vi "Simulator.vi"() -> ()   [LabVIEW 2018]
uses:
  Commands/Address.ctl
  <vilib>/FPGAPlugInAG/cRIO-9039/niLvFpga_Open_cRIO-9039.vi
  <vilib>/rvi/interface/common/dynamic/niFpgaDynamicAddResources.vi
  <vilib>/Utility/error.llb/Error Cluster From Error Code.vi
  <vilib>/rvi/errors/niLvFpgaAdjustHostInterfaceError.vi
  <vilib>/FPGAPlugInAG/Dynamic/niLvFpga_Close_Dynamic.vi
  <vilib>/rvi/interface/nirviOpenFPGA/nirviOpenFPGA.xnode
  FPGA Bitfiles/M1M3SupportSimulator.lvbitx
  <vilib>/rvi/interface/nirviMethod/nirviMethod.xnode
  <vilib>/rvi/interface/nirviCloseFPGA/nirviCloseFPGA.xnode
  <vilib>/rvi/errors/niLvFpgaMergeErrorWithErrorCode.vi
  <vilib>/FPGAPlugInAG/Dynamic/niLvFpga_WriteFifo_Dynamic.vi
  <vilib>/FPGAPlugInAG/Dynamic/niLvFpga_ReadFifo_Dynamic.vi
panel:
  out "E Instr":u64
  out "E Flags":u64 format="%04x"
  out "ERx":u64
  out "ETx":u64
  out "D Instr":u64
  out "D Flags":u64 format="%04x"
  out "DRx":u64
  out "DTx":u64
  out "C Instr":u64
  out "C Flags":u64 format="%04x"
  out "CRx":u64
  out "CTx":u64
  out "B Instr":u64
  out "B Flags":u64 format="%04x"
  out "BRx":u64
  out "BTx":u64
  out "String 5":string
  out "String 4":string
  out "String 3":string
  out "String 2":string
  out "String":string
  in  "Process Stop Button":bool
  out "A Instr":u64
  out "A Flags":u64 format="%04x"
  out "Error":string
  out "Loop count":dbl
  out "ARx":u64
  out "ATx":u64
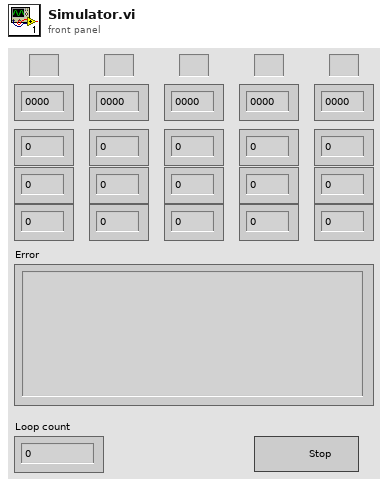
[diagram p1: front panel]
types:
  T1 = typedef "Address.ctl" = enum16{"ModbusA", "ModbusB", "ModbusC", "ModbusD", "ModbusE"}
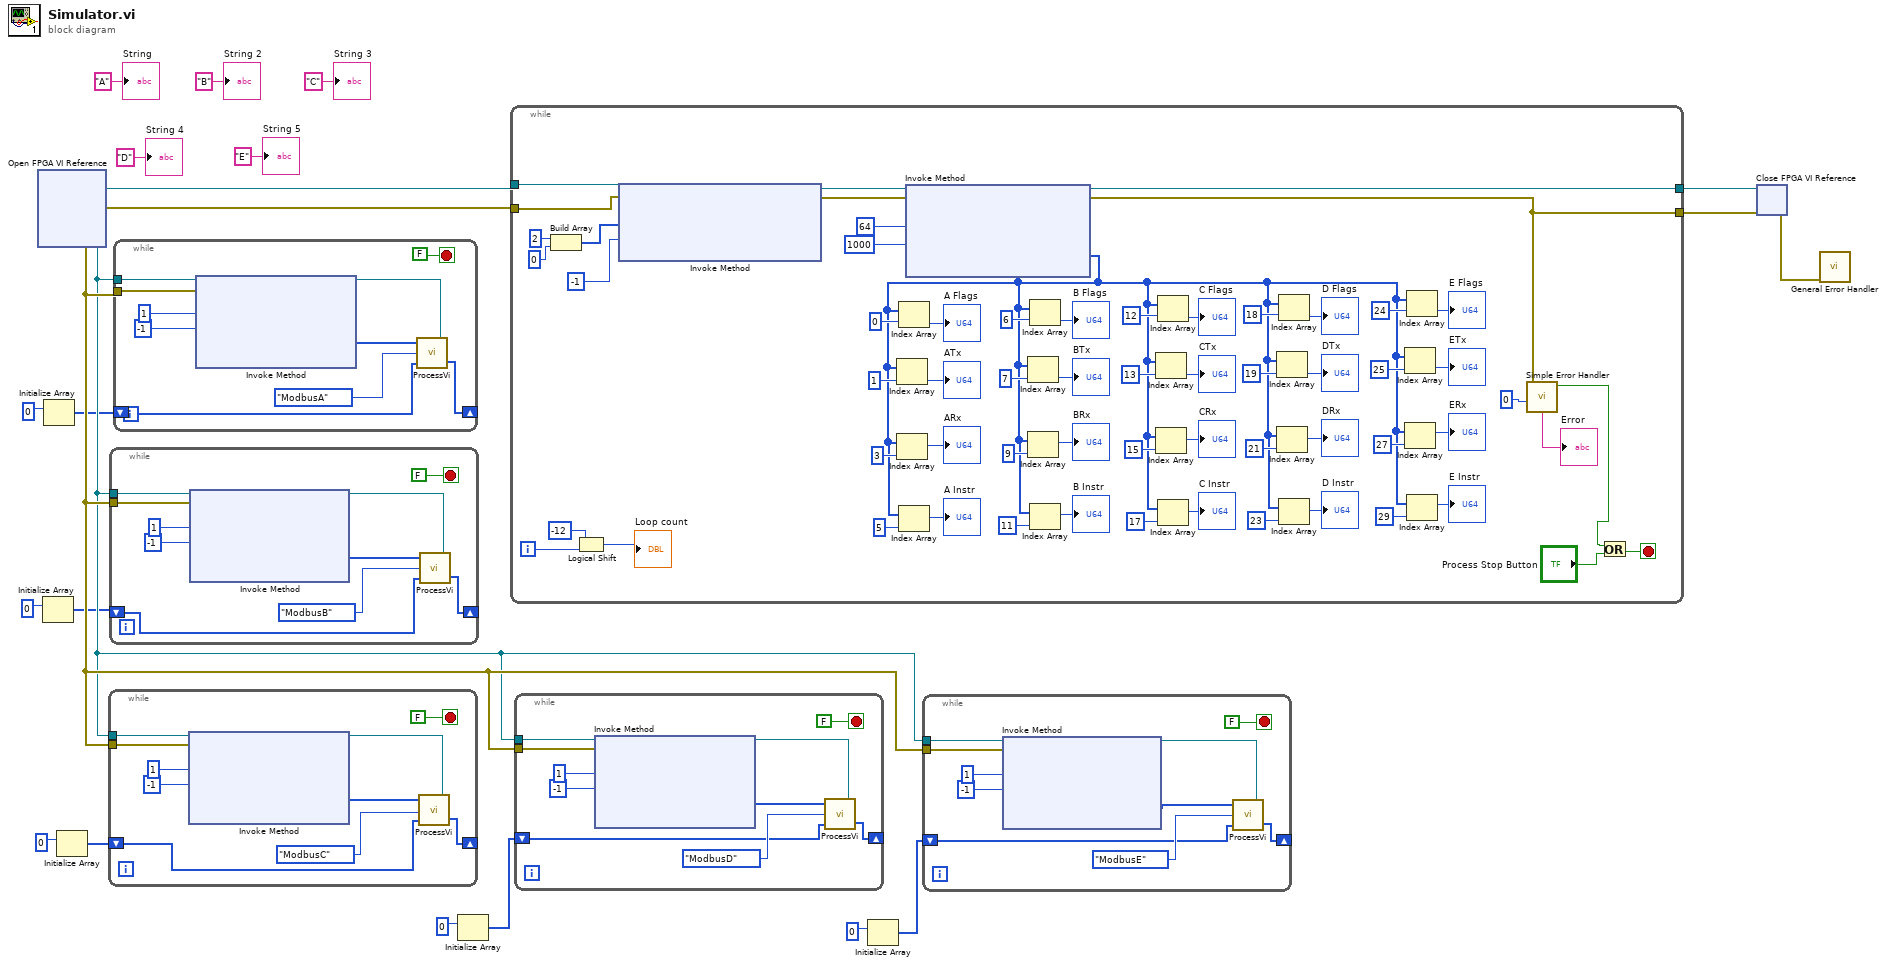
[diagram p0: block diagram]
diagram:
  n1 = xnode "Open FPGA VI Reference"() -> ("FPGA VI Reference Out"=w16:refnum<k20>, "error out"=w17:errorcluster)  [unwired: 2 in]
  n2 = Initialize Array(u8 0 ("element")) -> (w7:u8[])  [unwired: 1 in]
  n3 = Initialize Array(u8 0 ("element")) -> (w9:u8[])  [unwired: 1 in]
  n4 = Initialize Array(u8 0 ("element")) -> (w5:u8[])  [unwired: 1 in]
  n5 = while {
    tunnel: w17 -> [w26]
    tunnel: w16 -> [w25]
    shift-right: [w21] -> _
    shift-left: w5 -> [w22]
    stop <- FALSE stop-if-true
    n6 = xnode "Invoke Method"("FPGA VI Reference In"=w25, "error in"=w26, "Number of Elements"=u32 1, "Timeout (ms)"=-1) -> ("FPGA VI Reference Out"=w24:refnum<k20>, "Data"=w30:u16[])  [unwired: 2 out]
    n7 = call "ProcessVi.vi"("Refnum in"=w24, "Array In"=w22, "ModbusSend"=Address."ModbusC", "Data"=w30) -> ("Array out"=w21:u8[])
  }
  n8 = while {
    tunnel: w17 -> [w36]
    tunnel: w16 -> [w35]
    shift-right: [w31] -> _
    shift-left: w7 -> [w32]
    stop <- FALSE stop-if-true
    n9 = xnode "Invoke Method"("FPGA VI Reference In"=w35, "error in"=w36, "Number of Elements"=u32 1, "Timeout (ms)"=-1) -> ("FPGA VI Reference Out"=w34:refnum<k20>, "Data"=w40:u16[])  [unwired: 2 out]
    n10 = call "ProcessVi.vi"("Refnum in"=w34, "Array In"=w32, "ModbusSend"=Address."ModbusB", "Data"=w40) -> ("Array out"=w31:u8[])
  }
  n11 = while {
    tunnel: w17 -> [w45]
    tunnel: w16 -> [w44]
    shift-right: [w41] -> _
    shift-left: w9 -> [w42]
    stop <- FALSE stop-if-true
    n12 = xnode "Invoke Method"("FPGA VI Reference In"=w44, "error in"=w45, "Number of Elements"=u32 1, "Timeout (ms)"=-1) -> ("FPGA VI Reference Out"=w43:refnum<k20>, "Data"=w48:u16[])  [unwired: 2 out]
    n13 = call "ProcessVi.vi"("Refnum in"=w43, "Array In"=w42, "ModbusSend"=Address."ModbusA", "Data"=w48) -> ("Array out"=w41:u8[])
  }
  n14 = Initialize Array(u8 0 ("element")) -> (w3:u8[])  [unwired: 1 in]
  n15 = while {
    tunnel: w16 -> [w111]
    tunnel: [w98] -> w19
    tunnel: [w97] -> w18
    tunnel: w17 -> [w95]
    i -> [w53]
    stop <- w90 stop-if-true
    n16 = Build Array(u32 2 ("element"), u32 0 ("element")) -> (w109:u32[])
    n17 = Logical Shift(y=-12 ("x << y"), x=w53) -> (x << y=→"Loop count":i32)
    n18 = xnode "Invoke Method"("FPGA VI Reference In"=w111, "error in"=w95, "Data"=w109, "Timeout (ms)"=-1) -> ("FPGA VI Reference Out"=w106:refnum<k20>, "error out"=w105:errorcluster)  [unwired: 1 out]
    n19 = xnode "Invoke Method"("FPGA VI Reference In"=w106, "error in"=w105, "Number of Elements"=u32 64, "Timeout (ms)"=1000) -> ("FPGA VI Reference Out"=w98:refnum<k20>, "error out"=w97:errorcluster, "Data"=w56:u64[])  [unwired: 1 out]
    n20 = Index Array(array=w56, index=u64 1 ("element")) -> (element=→"ATx":u64)
    n21 = Index Array(array=w56, index=u64 3 ("element")) -> (element=→"ARx":u64)
    n22 = Index Array(array=w56, index=u64 0 ("element")) -> (element=→"A Flags":u64)
    n23 = Index Array(array=w56, index=u64 5 ("element")) -> (element=→"A Instr":u64)
    n24 = Index Array(array=w56, index=u64 7 ("element")) -> (element=→"BTx":u64)
    n25 = Index Array(array=w56, index=u64 9 ("element")) -> (element=→"BRx":u64)
    n26 = Index Array(array=w56, index=u64 6 ("element")) -> (element=→"B Flags":u64)
    n27 = Index Array(array=w56, index=u64 11 ("element")) -> (element=→"B Instr":u64)
    n28 = Index Array(array=w56, index=u64 13 ("element")) -> (element=→"CTx":u64)
    n29 = Index Array(array=w56, index=u64 15 ("element")) -> (element=→"CRx":u64)
    n30 = Index Array(array=w56, index=u64 12 ("element")) -> (element=→"C Flags":u64)
    n31 = Index Array(array=w56, index=u64 17 ("element")) -> (element=→"C Instr":u64)
    n32 = Index Array(array=w56, index=u64 19 ("element")) -> (element=→"DTx":u64)
    n33 = Index Array(array=w56, index=u64 21 ("element")) -> (element=→"DRx":u64)
    n34 = Index Array(array=w56, index=u64 18 ("element")) -> (element=→"D Flags":u64)
    n35 = Index Array(array=w56, index=u64 23 ("element")) -> (element=→"D Instr":u64)
    n36 = Index Array(array=w56, index=u64 25 ("element")) -> (element=→"ETx":u64)
    n37 = Index Array(array=w56, index=u64 27 ("element")) -> (element=→"ERx":u64)
    n38 = Index Array(array=w56, index=u64 24 ("element")) -> (element=→"E Flags":u64)
    n39 = Index Array(array=w56, index=u64 29 ("element")) -> (element=→"E Instr":u64)
    n40 = call <vilib>:"Simple Error Handler.vi"("type of dialog (OK msg:1)"=0, "error in (no error)"=w97) -> ("error?"=w54:bool, "message"=→"Error":string)  [unwired: 3 in, 3 out]
    n41 = Or(x=w54, y="Process Stop Button") -> (x .or. y?=w90:bool)
  }
  n42 = while {
    tunnel: w17 -> [w117]
    tunnel: w16 -> [w116]
    shift-right: [w112] -> _
    shift-left: w3 -> [w113]
    stop <- FALSE stop-if-true
    n43 = xnode "Invoke Method"("FPGA VI Reference In"=w116, "error in"=w117, "Number of Elements"=u32 1, "Timeout (ms)"=-1) -> ("FPGA VI Reference Out"=w115:refnum<k20>, "Data"=w121:u16[])  [unwired: 2 out]
    n44 = call "ProcessVi.vi"("Refnum in"=w115, "Array In"=w113, "ModbusSend"=Address."ModbusD", "Data"=w121) -> ("Array out"=w112:u8[])
  }
  n45 = Initialize Array(u8 0 ("element")) -> (w1:u8[])  [unwired: 1 in]
  n46 = while {
    tunnel: w17 -> [w127]
    tunnel: w16 -> [w126]
    shift-right: [w122] -> _
    shift-left: w1 -> [w123]
    stop <- FALSE stop-if-true
    n47 = xnode "Invoke Method"("FPGA VI Reference In"=w126, "error in"=w127, "Number of Elements"=u32 1, "Timeout (ms)"=-1) -> ("FPGA VI Reference Out"=w125:refnum<k20>, "Data"=w131:u16[])  [unwired: 2 out]
    n48 = call "ProcessVi.vi"("Refnum in"=w125, "Array In"=w123, "ModbusSend"=Address."ModbusE", "Data"=w131) -> ("Array out"=w122:u8[])
  }
  n49 = xnode "Close FPGA VI Reference"("FPGA VI Reference In"=w19, "error in"=w18) -> ("error out"=w20:errorcluster)
  n50 = call <vilib>:"General Error Handler.vi"("error in (no error)"=w20) -> ()  [unwired: 10 in, 5 out]
  "String" <- "A"
  "String 2" <- "B" ("String 2")
  "String 3" <- "C" ("String 3")
  "String 4" <- "D" ("String 4")
  "String 5" <- "E" ("String 5")
